vi "TC_messenger.vi"() -> ()   [LabVIEW 2017]
panel:
  out "program version":string
  out "Last update":string
  in  "Leidon IP address":string="127.0.0.1"
  out "Server connected?":bool
  out "Msg out":string
  out "Msg In":string
  out "Client connected?":bool
  # "tcp-visa-server\nfor TC program"
  # "port 6340"
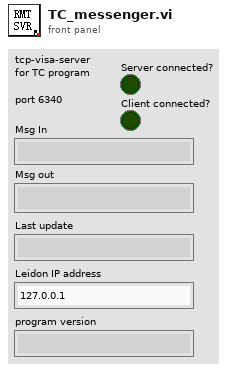
[diagram p1: front panel]
types:
  T1 = enum16{"Standard", "Buffered", "CRLF", "Immediate"}
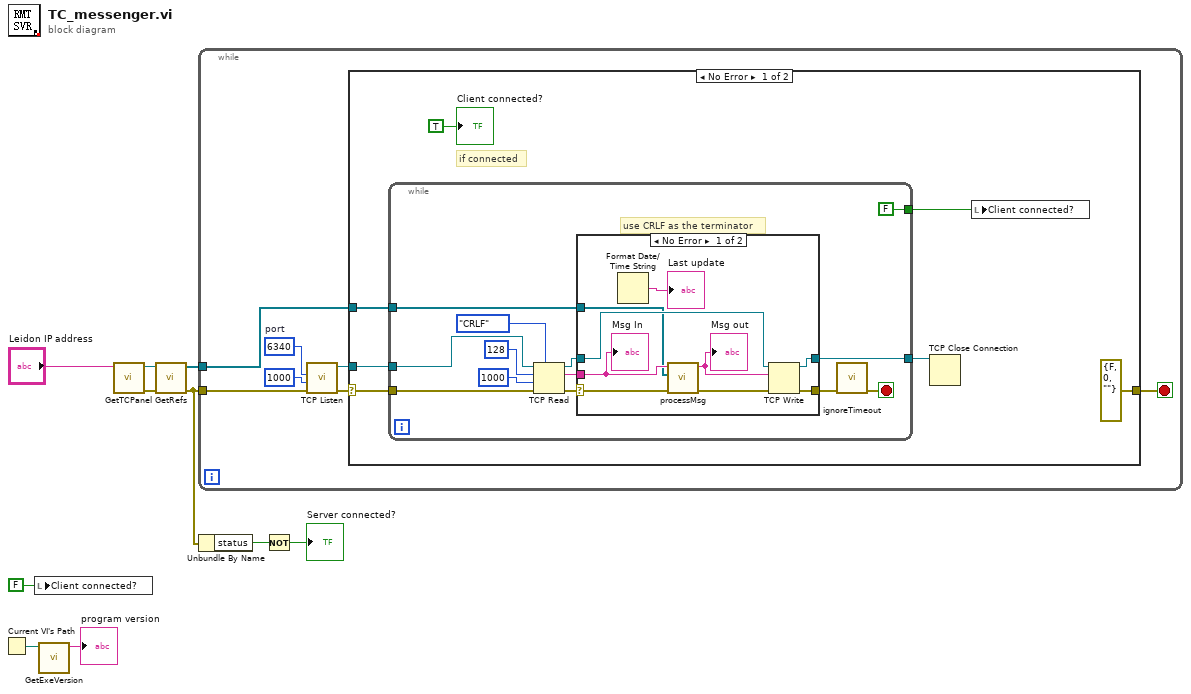
[diagram p0: block diagram]
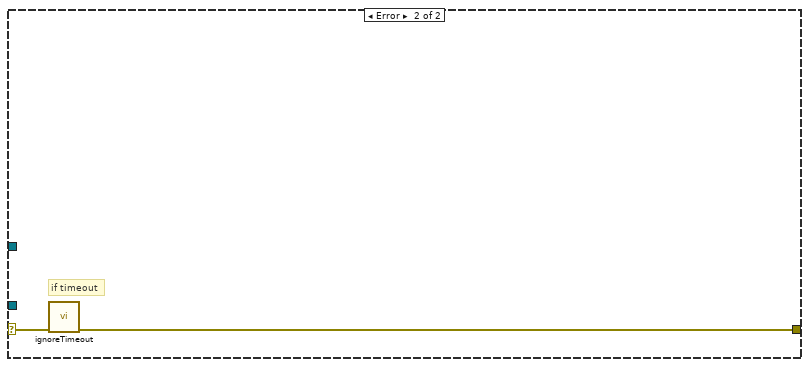
[diagram p3: hidden frame]
diagram:
  n1 = Current VI's Path() -> (path=w6:path)
  n2 = local write "Client connected?"(FALSE ("remote?")) -> ()
  n3 = call "GetExeVersion.vi"("路径"=w6) -> ("Version of Executable"=→"program version":string)  [unwired: 10 out]
  n4 = call "GetTCPanel.vi"("ip"="Leidon IP address") -> ("error out"=w4:errorcluster, "panel"=w1:refnum<vi>)  [unwired: 1 in, 6 out]
  n5 = call "GetRefs.vi"("error in (no error)"=w4, "panel"=w1) -> ("error out"=w3:errorcluster, "Refs"=w2:refnum<vi>[])  [unwired: 8 in]
  n6 = while {
    tunnel: w2 -> [w12]
    tunnel: w3 -> [w11]
    stop <- w14 stop-if-true
    w17 = u16 6340  # port
    n7 = call <vilib>:"TCP Listen.vi"("error in (no error)"=w11, "timeout ms (wait forever: -1)"=1000, "port"=w17) -> ("error out"=w13:errorcluster, "connection ID"=w16:refnum<k5>)  [unwired: 1 in, 6 out]
    n8 = case shown="No Error" w13 {
      selector: w13 -> [w20 w49]
      tunnel: w16 -> [w24 _]
      tunnel: [errorcluster {"status"=FALSE, "code"=0, "source"=""} ("error out") w50] -> w14
      tunnel: w12 -> [w18 _]
      frame No Error {
        # "if connected"
        n9 = while {
          tunnel: w24 -> [w30]
          tunnel: [w37] -> w23
          tunnel: w20 -> [w33]
          tunnel: [FALSE ("remote")] -> w21
          tunnel: w18 -> [w26]
          stop <- w34 stop-if-true
          # "use CRLF as the terminator"
          n10 = TCP Read(connection ID=w30, bytes to read=128, error in (no error)=w33, 7:T1."CRLF" ("mode (standard)"), 9:1000 ("timeout ms (25000)")) -> (connection ID out=w28:refnum<k5>, data out=w27:string, error out=w25:errorcluster)
          n11 = case shown="No Error" w25 {
            selector: w25 -> [w40 w48]
            tunnel: [w46 w47] -> w37
            tunnel: [w45 w48] -> w35
            tunnel: w28 -> [w44 w47]
            tunnel: w27 -> [w43 _]
            tunnel: w26 -> [w38 _]
            frame No Error {
              n12 = Format Date/Time String() -> (date/time string=→"Last update":string)  [unwired: 3 out]
              n13 = call "processMsg.vi"("error in (no error)"=w40, "Refs"=w38, "Msg in"=w43) -> ("error out"=w41:errorcluster, "Msg out"=w42:string)  [unwired: 7 out]
              "Msg out" <- w42
              n14 = TCP Write(connection ID=w44, data in=w42, error in (no error)=w41) -> (connection ID out=w46:refnum<k5>, error out=w45:errorcluster)  [unwired: 2 out]
              "Msg In" <- w43
            }
            frame Error {
            }
          }
          n15 = call "ignoreTimeout.vi"("error in (no error)"=w35) -> ("error out"=w34:errorcluster)  [unwired: 10 out]
        }
        n16 = TCP Close Connection(connection ID=w23) -> ()  [unwired: 1 in, 3 out]
        n17 = local write "Client connected?"(w21) -> ()
        "Client connected?" <- TRUE ("remote")
      }
      frame Error {
        # "if timeout"
        n18 = call "ignoreTimeout.vi"("error in (no error)"=w49) -> ("error out"=w50:errorcluster)  [unwired: 10 out]
      }
    }
  }
  n19 = Unbundle By Name(w3) -> ("status"=w8:bool)
  n20 = Not(x=w8) -> (.not. x?=→"Server connected?":bool)
